vi "Fill XLSX Multicells.vi"(8 "error in (no error)":errorcluster, 10 "Cell Span":T1(array[cluster]), 11 "Array in":string[][](array[string])) -> (0 "error out":errorcluster, 3 "Array out":string[][](array[string]))   [LabVIEW 2021, in "Files.lvlib"]
doc: "Fills table with copies of the single-copy value of multicell-spanning super-cell."
uses:
  Files.lvlib
panel:
  out "Multicell Spans":i32[](array[numeric])
  # "see the AlliGator License on the block diagram (Ctrl+E or Window:Show Block Diagram)"
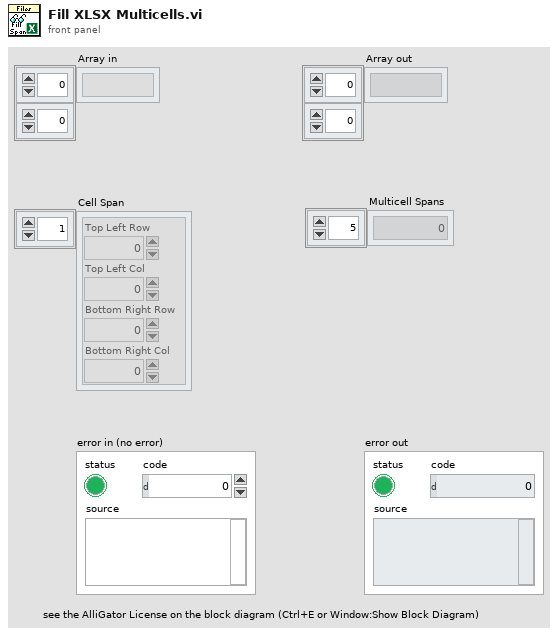
[diagram p1: front panel]
types:
  T1 = cluster{"Top Left Row":i32, "Top Left Col":i32, "Bottom Right Row":i32, "Bottom Right Col":i32}[]
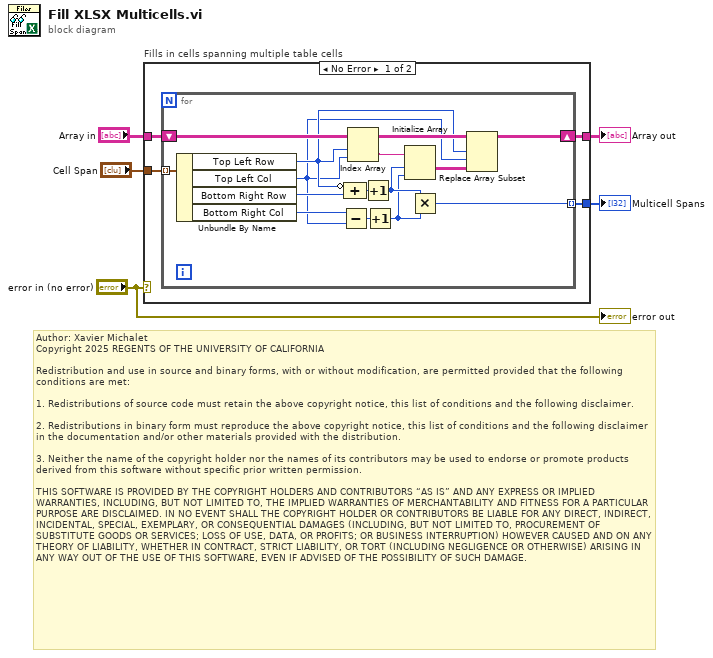
[diagram p0: block diagram]
diagram:
  # "Author: Xavier Michalet\nCopyright 2025 REGENTS OF THE UNIVERSITY OF CALIFORNIA\n\nRedistribution and use in source and binary forms, with or without modification, are permitted provided that the following conditions are met:\n\n1. Redistributions of source code must retain the above copyright notice, this list of conditions and the following disclaimer.\n\n2. Redistributions in binary form must reproduce the above copyright notice, this list of conditions and the following disclaimer in the documentation and/or other materials provided with the distribution.\n\n3. Neither the name of the copyright holder nor the names of its contributors may be used to endorse or promote products derived from this software without specific prior written permission.\n\nTHIS SOFTWARE IS PROVIDED BY THE COPYRIGHT HOLDERS AND CONTRIBUTORS “AS IS” AND ANY EXPRESS OR IMPLIED WARRANTIES, INCLUDING, BUT NOT LIMITED TO, THE IMPLIED WARRANTIES OF MERCHANTABILITY AND FITNESS FOR A PARTICULAR PURPOSE ARE DISCLAIMED. IN NO EVENT SHALL THE COPYRIGHT HOLDER OR CONTRIBUTORS BE LIABLE FOR ANY DIRECT, INDIRECT, INCIDENTAL, SPECIAL, EXEMPLARY, OR CONSEQUENTIAL DAMAGES (INCLUDING, BUT NOT LIMITED TO, PROCUREMENT OF SUBSTITUTE GOODS OR SERVICES; LOSS OF USE, DATA, OR PROFITS; OR BUSINESS INTERRUPTION) HOWEVER CAUSED AND ON ANY THEORY OF LIABILITY, WHETHER IN CONTRACT, STRICT LIABILITY, OR TORT (INCLUDING NEGLIGENCE OR OTHERWISE) ARISING IN ANY WAY OUT OF THE USE OF THIS SOFTWARE, EVEN IF ADVISED OF THE POSSIBILITY OF SUCH DAMAGE."
  n1 = case "Fills in cells spanning multiple table cells" shown="No Error" "error in (no error)" {
    tunnel: "Array in" -> [w9 w24]
    tunnel: [w8 w24] -> w4
    tunnel: "Cell Span" -> [w7 _]
    tunnel: [w6 _] -> w1
    frame No Error {
      n2 = for {
        shift-right: [w19] -> w8
        shift-left: w9 -> [w20]
        tunnel: w7 -> [w23] mode=indexing
        tunnel: [w10] -> w6 mode=indexing
        n3 = Unbundle By Name(w23) -> ("Top Left Row"=w14:i32, "Top Left Col"=w13:i32, "Bottom Right Row"=w22:i32, "Bottom Right Col"=w21:i32)
        n4 = Subtract(x=w21, y=w13) -> (x-y=w16:i32)
        n5 = Compound Arithmetic op=ADD(invert w14, w22) -> (w17:i32)
        n6 = Index Array(array=w20, index (row)=w14, index (col)=w13) -> (element=w18:string)
        n7 = Increment(x=w17) -> (x+1=w12:i32)
        n8 = Increment(x=w16) -> (x+1=w11:i32)
        n9 = Initialize Array(w18, w12, w11) -> (w15:string[][])
        n10 = Multiply(x=w12, y=w11) -> (x*y=w10:i32)
        n11 = Replace Array Subset(array=w20, new element=w15, index (row)=w14, index (col)=w13) -> (w19:string[][])
      }
    }
    frame Error {
    }
  }
  "Array out" <- w4
  "Multicell Spans" <- w1
  "error out" <- "error in (no error)"
